vi "CRYGet Freq Bit Array.vi"(10 "Boolean":bool=TRUE, 11 "Device Infor":T1) -> (0 "MaxFreq":u32, 1 "MinFreq":u32, 2 "Bit Depth":cluster{"String":string, "Value":ext}[](array[cluster]), 3 "Samplein Rate":cluster{"String":string, "Value":ext}[](array[cluster]))   [LabVIEW 2013]
panel:
  # "Get Frequency Bit Array"
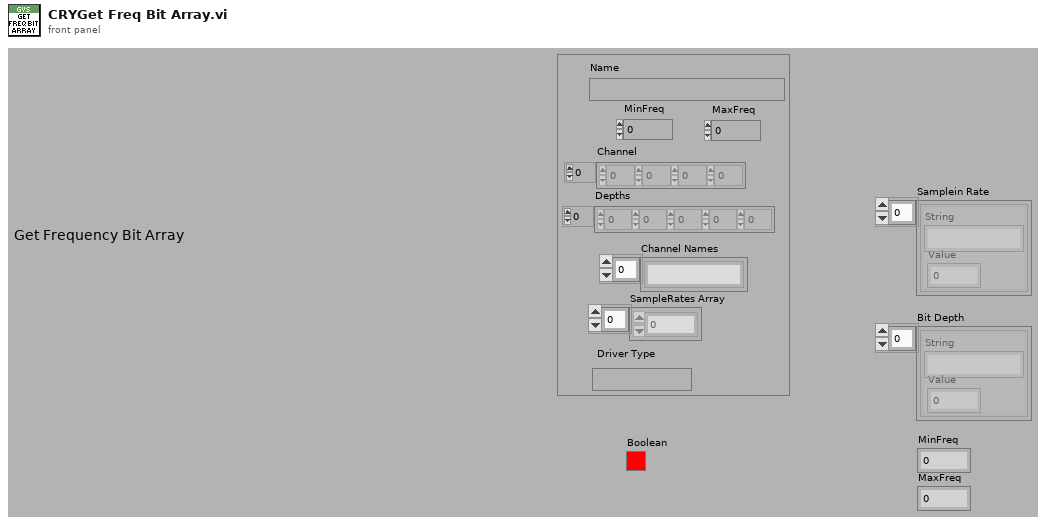
[diagram p1: front panel]
types:
  T1 = cluster{"Name":string, "MinFreq":dbl, "MaxFreq":dbl, "Channel":i32[], "Depths":i32[], "Channel Names":string[], "SampleRates Array":dbl[], "Driver Type":string}
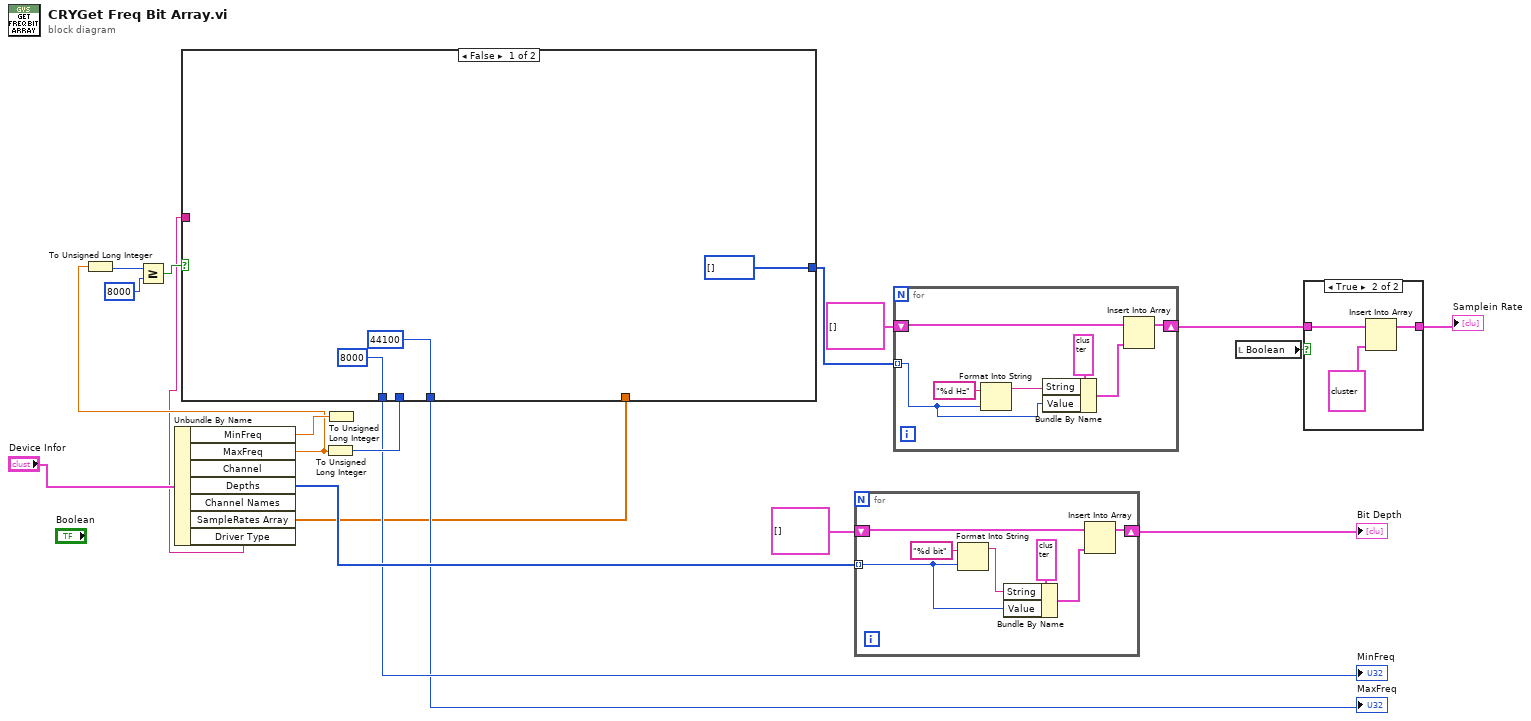
[diagram p0: block diagram]
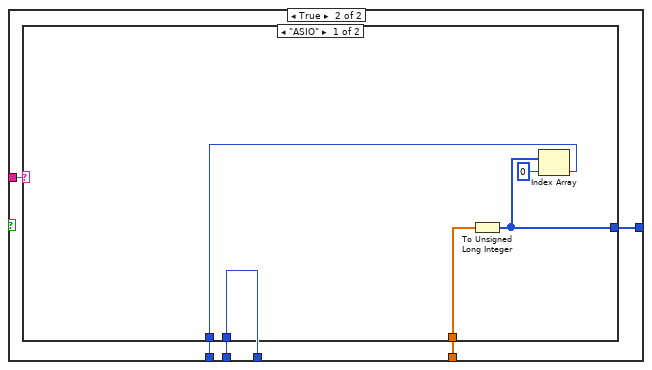
[diagram p2: hidden frame]
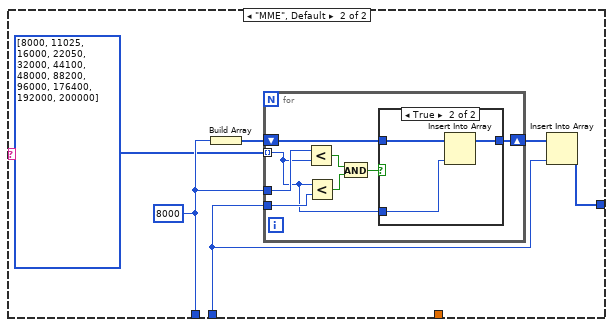
[diagram p3: hidden frame]
diagram:
  n1 = Unbundle By Name("Device Infor") -> ("MinFreq"=w16:dbl, "MaxFreq"=w8:dbl, "Depths"=w11:i32[], "SampleRates Array"=w1:dbl[], "Driver Type"=w2:string)  [unwired: 2 out]
  n2 = To Unsigned Long Integer(number=w8) -> (unsigned 32bit integer=w6:u32)
  n3 = Greater Or Equal?(x=w6, y=u32 8000) -> (x >= y?=w5:bool)
  n4 = To Unsigned Long Integer(number=w8) -> (unsigned 32bit integer=w13:u32)
  n5 = case shown="False" w5 {
    tunnel: [u32[] [] w27] -> w14
    tunnel: w13 -> [_ w25]
    tunnel: [u32 8000 ("unsigned 32bit integer") w26] -> w10
    tunnel: [u32 44100 w25] -> w4
    tunnel: w2 -> [_ w24]
    tunnel: w1 -> [_ w23]
    frame False {
    }
    frame True {
      n6 = case shown="\"ASIO\"" w24 {
        tunnel: [w30 w37] -> w27
        tunnel: [w28 w36] -> w26
        tunnel: w25 -> [_ w32]
        tunnel: w23 -> [w31 _]
        frame "ASIO" {
          n7 = To Unsigned Long Integer(number=w31) -> (unsigned 32bit integer=w30:u32[])
          n8 = Index Array(array=w30, index=0) -> (element=w28:u32)
        }
        frame "MME", Default {
          w36 = u32 8000 ("unsigned 32bit integer")
          n9 = Build Array(w36) -> (w34:u32[])
          n10 = for {
            tunnel: w32 -> [w40]
            tunnel: w36 -> [w39]
            tunnel: u32[] [8000, 11025, 16000, 22050, 32000, 44100, 48000, 88200, 96000, 176400, 192000, 200000] -> [w38] mode=indexing
            shift-right: [w42] -> w33
            shift-left: w34 -> [w41]
            n11 = Less?(x=w39, y=w38) -> (x < y?=w45:bool)
            n12 = Less?(x=w38, y=w40) -> (x < y?=w44:bool)
            n13 = And(x=w45, y=w44) -> (x .and. y?=w43:bool)
            n14 = case shown="True" w43 {
              tunnel: [w46 w49] -> w42
              tunnel: w41 -> [w46 w48]
              tunnel: w38 -> [_ w47]
              frame False {
              }
              frame True {
                n15 = Insert Into Array(array=w48, new element=w47) -> (w49:u32[])  [unwired: 1 in]
              }
            }
          }
          n16 = Insert Into Array(array=w33, new element=w32) -> (w37:u32[])  [unwired: 1 in]
        }
      }
    }
  }
  "MinFreq" <- w10
  "MaxFreq" <- w4
  n17 = To Unsigned Long Integer(number=w16) -> ()  [unwired: 1 out]
  n18 = for {
    tunnel: w11 -> [w51] mode=indexing
    shift-right: [w56] -> w9
    shift-left: cluster{"String":string, "Value":ext}[] [] -> [w55]
    n19 = Format Into String(format string="%d bit", w51) -> (resulting string=w53:string)  [unwired: 2 in, 1 out]
    n20 = Bundle By Name(cluster=cluster{"String":string, "Value":ext} {"String"="", "Value"=0.0}, "String"=w53, "Value"=w51) -> (w50:cluster{"String":string, "Value":ext})
    n21 = Insert Into Array(array=w55, new element=w50) -> (w56:cluster{"String":string, "Value":ext}[])  [unwired: 1 in]
  }
  "Bit Depth" <- w9
  n22 = for {
    shift-right: [w63] -> w18
    shift-left: cluster{"String":string, "Value":ext}[] [] -> [w62]
    tunnel: w14 -> [w57] mode=indexing
    n23 = Format Into String(format string="%d Hz", w57) -> (resulting string=w60:string)  [unwired: 2 in, 1 out]
    n24 = Bundle By Name(cluster=cluster{"String":string, "Value":ext} {"String"="", "Value"=0.0}, "String"=w60, "Value"=w57) -> (w58:cluster{"String":string, "Value":ext})
    n25 = Insert Into Array(array=w62, new element=w58) -> (w63:cluster{"String":string, "Value":ext}[])  [unwired: 1 in]
  }
  n26 = local read "Boolean"() -> (w12:bool)
  n27 = case shown="True" w12 {
    tunnel: w18 -> [w64 w67]
    tunnel: [w64 w65] -> w17
    frame False {
    }
    frame True {
      n28 = Insert Into Array(array=w67, new element=cluster{"String":string, "Value":ext} {"String"="User", "Value"=0.0} ("new element/subarray")) -> (w65:cluster{"String":string, "Value":ext}[])  [unwired: 1 in]
    }
  }
  "Samplein Rate" <- w17
